vi "转换元素.vi"(1 "空的位置":cluster{"x":i32, "y":i32}, 2 "按键位置":cluster{"x":i32, "y":i32}, 3 "输入数组":dbl[](array[numeric])) -> (0 "输出数组":dbl[](array[numeric]))   [LabVIEW 2009]
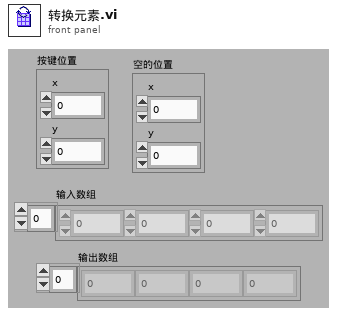
[diagram p1: front panel]
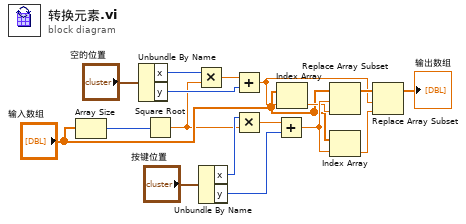
[diagram p0: block diagram]
diagram:
  n1 = Array Size(array="输入数组") -> (size(s)=w2:i32)
  n2 = Unbundle By Name("空的位置") -> ("x"=w14:i32, "y"=w10:i32)
  n3 = Square Root(x=w2) -> (sqrt(x)=w1:dbl)
  n4 = Multiply(x=w14, y=w1) -> (x*y=w11:dbl)
  n5 = Unbundle By Name("按键位置") -> ("x"=w15:i32, "y"=w12:i32)
  n6 = Add(x=w11, y=w10) -> (x+y=w6:dbl)
  n7 = Multiply(x=w15, y=w1) -> (x*y=w13:dbl)
  n8 = Add(x=w13, y=w12) -> (x+y=w9:dbl)
  n9 = Index Array(array="输入数组", index=w6) -> (element=w8:dbl)
  n10 = Replace Array Subset(array="输入数组", new element=w8, index=w9) -> (w7:dbl[])
  n11 = Index Array(array="输入数组", index=w9) -> (element=w5:dbl)
  n12 = Replace Array Subset(array=w7, new element=w5, index=w6) -> (→"输出数组":dbl[])
